vi "servo_plate_heater.vi"() -> ()   [LabVIEW 2015]
uses:
  <vilib>/addons/control/pid/pid.llb/PID Advanced (DBL).vi
  <vilib>/addons/control/pid/NI_PID_pid.lvlib
panel:
  in  "PID Gains":T1={"proportional gain (Kc)"=1.3979250340642948, "integral time (Ti, min)"=2.9580260274160532, "derivative time (Td, min)"=0.46155392250462524} {"derivative time (Td, min)" format="%#.6g"; "integral time (Ti, min)" format="%#.6g"; "proportional gain (Kc)" format="%#.6g"}
  in  "dt (s)":dbl=1.0 format="%.3f"
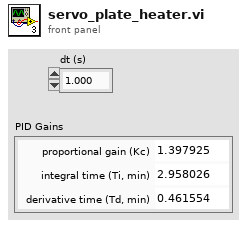
[diagram p1: front panel]
types:
  T1 = cluster{"proportional gain (Kc)":dbl, "integral time (Ti, min)":dbl, "derivative time (Td, min)":dbl}
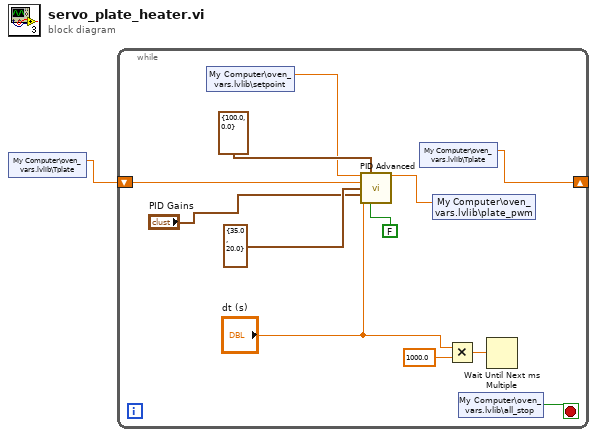
[diagram p0: block diagram]
diagram:
  n1 = shared-variable "My Computer\\oven_vars.lvlib\\Tplate"() -> (w1:dbl)  [unwired: 1 in, 1 out]
  n2 = while {
    shift-right: [w5] -> _
    shift-left: w1 -> [w7]
    stop <- w4 stop-if-true
    n3 = shared-variable "My Computer\\oven_vars.lvlib\\setpoint"() -> (w3:dbl)  [unwired: 1 in, 1 out]
    n4 = call-poly <vilib>:"PID Advanced.vi"("setpoint"=w3, "output range"=cluster{"output high":dbl, "output low":dbl} {"output high"=100.0, "output low"=0.0}, "process variable"=w7, "setpoint range"=cluster{"setpoint high":dbl, "setpoint low":dbl} {"setpoint high"=35.0, "setpoint low"=20.0}, "PID gains"="PID Gains", "dt (s)"="dt (s)", "reinitialize? (F)"=FALSE) -> ("output"=w6:dbl)  [unwired: 7 in, 1 out]
    n5 = shared-variable "My Computer\\oven_vars.lvlib\\Tplate"() -> (w5:dbl)  [unwired: 1 in, 1 out]
    n6 = shared-variable "My Computer\\oven_vars.lvlib\\plate_pwm"(w6) -> ()  [unwired: 1 in, 1 out]
    n7 = Multiply(x="dt (s)", y=1000.0) -> (x*y=w10:dbl)
    n8 = shared-variable "My Computer\\oven_vars.lvlib\\all_stop"() -> (w4:bool)  [unwired: 1 in, 1 out]
    n9 = Wait Until Next ms Multiple(millisecond multiple=w10) -> ()  [unwired: 1 out]
  }
